vi "Launch New Chat Window.vi"(8 "error in (no error)":errorcluster, 11 "Server in":refnum<class "Server.lvclass">) -> (0 "error out":errorcluster, 3 "Server out":refnum<class "Server.lvclass">)   [LabVIEW 2020, in "Server.lvlib" / "Server.lvclass"]
uses:
  Server.lvclass
  C:/Program Files/National Instruments/LabVIEW 2020/vi.lib/ActorFramework/Actor/Actor.lvclass
  Chat Window Model/Chat Window Model/Chat Window Model.lvclass
  <vilib>/ActorFramework/Message Enqueuer/Message Enqueuer.lvclass
  Chat Window Model/Chat Window Model/Chat Window Model.lvclass/Chat Window Model.ctl
  <vilib>/ActorFramework/Actor/Actor.lvclass/Actor.ctl
  <vilib>/ActorFramework/Message Enqueuer/Message Enqueuer.lvclass/Message Enqueuer.ctl
  Server.lvclass/Server.ctl
  Server Messages/Enable Controls Msg/Enable Controls Msg.lvclass/Enable Controls Msg.ctl
  Chat Window Model/Chat Window Model Messages/Update Status Log Msg/Update Status Log Msg.lvclass/Update Status Log Msg.ctl
  Chat Window Model/Chat Window Model Messages/Update Online List Msg/Update Online List Msg.lvclass/Update Online List Msg.ctl
  SubPanel-Actor-Framework-master/Event-Source-Actor/Source/Template Source/Event Source Messages/Register For Event Msg/Register For Event Msg.lvclass/Register For Event Msg.ctl
  <vilib>/ActorFramework/Message Enqueuer/Init from Existing Queue.vi
  <vilib>/ActorFramework/Message Enqueuer/Enqueue.vi
  Server Messages/Enable Controls Msg/Enable Controls Msg.lvclass
  C:/Program Files/National Instruments/LabVIEW 2020/vi.lib/ActorFramework/Message/Message.lvclass
  Chat Window Model/Chat Window Model Messages/Update Status Log Msg/Update Status Log Msg.lvclass
  Chat Window Model/Chat Window Model Messages/Update Online List Msg/Update Online List Msg.lvclass
  SubPanel-Actor-Framework-master/Event-Source-Actor/Source/Template Source/Event Source Messages/Register For Event Msg/Register For Event Msg.lvclass
  <vilib>/ActorFramework/Message Priority Queue/Priority Enqueue.vi
  <vilib>/ActorFramework/Actor/Actor.lvclass
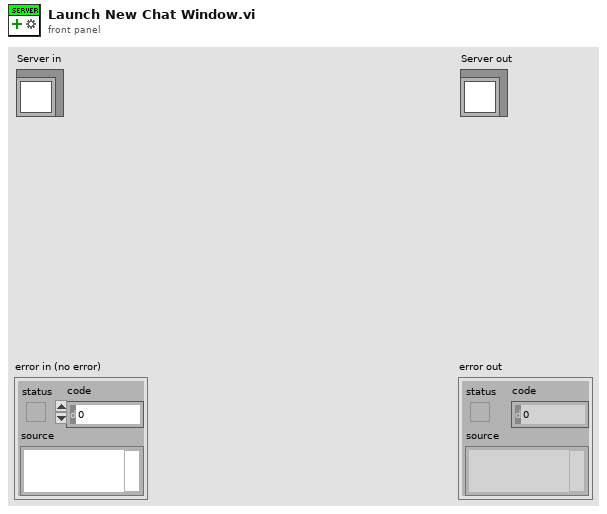
[diagram p1: front panel]
types:
  T1 = cluster{"Enqueuer":refnum<class "Message Enqueuer.lvclass">, "Status":string}
  T2 = enum8{"Enabled", "Disabled", "Disabled and Grayed Out"}
  T3 = map{string, cluster{"Enqueuer":refnum<class "Message Enqueuer.lvclass">, "Status":string}}
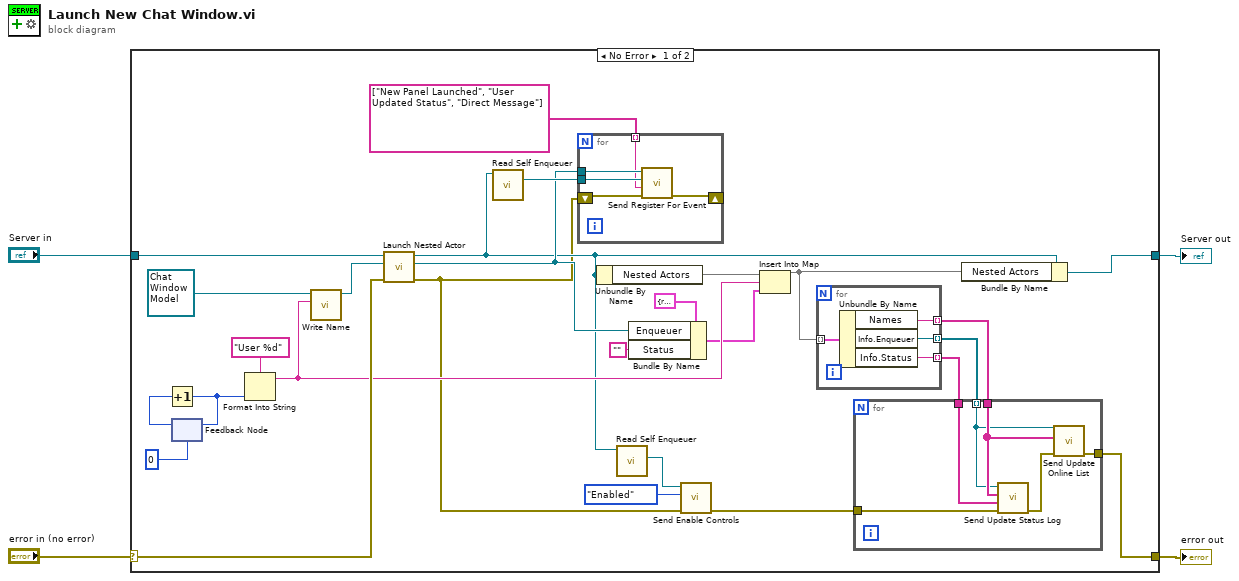
[diagram p0: block diagram]
diagram:
  n1 = case shown="No Error" "error in (no error)" {
    selector: "error in (no error)" -> [w30 w48]
    tunnel: [w23 w48] -> w3
    tunnel: [w24 w47] -> w1
    tunnel: "Server in" -> [w31 w47]
    frame No Error {
      n2 = feedback #1(0) -> (w27:i32)
      n3 = Increment(x=w27) -> (x+1=w25:i32)
      n4 = feedback-in #1(w25) -> ()
      n5 = Format Into String(format string="User %d", w25) -> (resulting string=w18:string)  [unwired: 2 in, 1 out]
      n6 = call "Write Name.vi"("Name"=w18, "Chat Window Model in"=refnum<class "Chat Window Model.lvclass"> refnum ("Chat Window Model.lvlib:Chat Window Model.lvclass")) -> ("Chat Window Model out"=w29:refnum<class "Chat Window Model.lvclass">)  [unwired: 8 in, 1 out]
      n7 = call <vilib>:"Launch Nested Actor.vi"("error in (no error)"=w30, "Nested Actor"=w29, "Caller Actor in"=w31) -> ("error out"=w5:errorcluster, "Nested Actor's Enqueuer"=w7:refnum<class "Message Enqueuer.lvclass">, "Caller Actor out"=w6:refnum<class "Server.lvclass">)  [unwired: 6 in]
      n8 = call <vilib>:"Read Self Enqueuer.vi"("Actor"=w6) -> ("Self Enqueuer"=w9:refnum<class "Message Enqueuer.lvclass">)  [unwired: 10 in]
      n9 = for {
        tunnel: w7 -> [w36]
        tunnel: w9 -> [w35]
        shift-right: [w33] -> _
        shift-left: w5 -> [w34]
        tunnel: string[] ["New Panel Launched", "User Updated Status", "Direct Message"] -> [w32] mode=indexing
        n10 = call "Send Register For Event.vi"("error in"=w34, "Event Name"=w32, "Registrant Enq"=w35, "Message Enqueuer"=w36) -> ("error out"=w33:errorcluster)  [unwired: 6 in, 1 out]
      }
      n11 = Unbundle By Name(w6) -> ("Nested Actors"=w19:T3)
      n12 = call <vilib>:"Read Self Enqueuer.vi"("Actor"=w6) -> ("Self Enqueuer"=w21:refnum<class "Message Enqueuer.lvclass">)  [unwired: 10 in]
      n13 = Bundle By Name(cluster=T1 {"Enqueuer"=refnum, "Status"=""} ("value"), "Enqueuer"=w7, "Status"="") -> (w15:T1)
      n14 = call "Send Enable Controls.vi"("error in (no error)"=w5, "Disabled"=T2."Enabled", "Message Enqueuer in"=w21) -> ("error out"=w22:errorcluster)  [unwired: 7 in, 1 out]
      n15 = Insert Into Map(map in=w19, key=w18, value=w15) -> (map out=w14:T3)  [unwired: 2 out]
      n16 = for {
        tunnel: [w39] -> w13 mode=indexing
        tunnel: w14 -> [w40] mode=indexing
        tunnel: [w38] -> w12 mode=indexing
        tunnel: [w37] -> w11 mode=indexing
        n17 = Unbundle By Name(w40) -> ("Names"=w39:string, "Info.Enqueuer"=w38:refnum<class "Message Enqueuer.lvclass">, "Info.Status"=w37:string)
      }
      n18 = for {
        tunnel: [w45] -> w23
        tunnel: w22 -> [w44]
        tunnel: w13 -> [w43]
        tunnel: w12 -> [w42] mode=indexing
        tunnel: w11 -> [w41]
        n19 = call "Send Update Status Log.vi"("error in (no error)"=w44, "Status List"=w41, "Names"=w43, "Message Enqueuer in"=w42) -> ("error out"=w46:errorcluster)  [unwired: 6 in, 1 out]
        n20 = call "Send Update Online List.vi"("error in (no error)"=w46, "Online Users"=w43, "Message Enqueuer in"=w42) -> ("error out"=w45:errorcluster)  [unwired: 7 in, 1 out]
      }
      n21 = Bundle By Name(cluster=w6, "Nested Actors"=w14) -> (w24:refnum<class "Server.lvclass">)
    }
    frame Error {
    }
  }
  "error out" <- w3
  "Server out" <- w1
